vi "VISATCP组合选择发送.vi"(0 "IP":string, 1 "数据发送通道":enum16{"TCP", "VISA"}(ring), 2 "命令":string(combo), 5 "PORT":string, 7 "VISA resource name":refnum<visa-resource-name> caption="VISA资源名称", 9 "baud rate":u32=115200 caption="波特率(115200)", 11 "error in (no error)":errorcluster caption="错误输入（无错误）", 12 "写入缓冲区":string) -> (4 "连接ID":refnum<k5>, 6 "VISA resource name 2":refnum<visa-resource-name>, 13 "读取缓冲区":string, 15 "错误输出":errorcluster)   [LabVIEW 2016, in "数据传输系统-03.lvlib"]
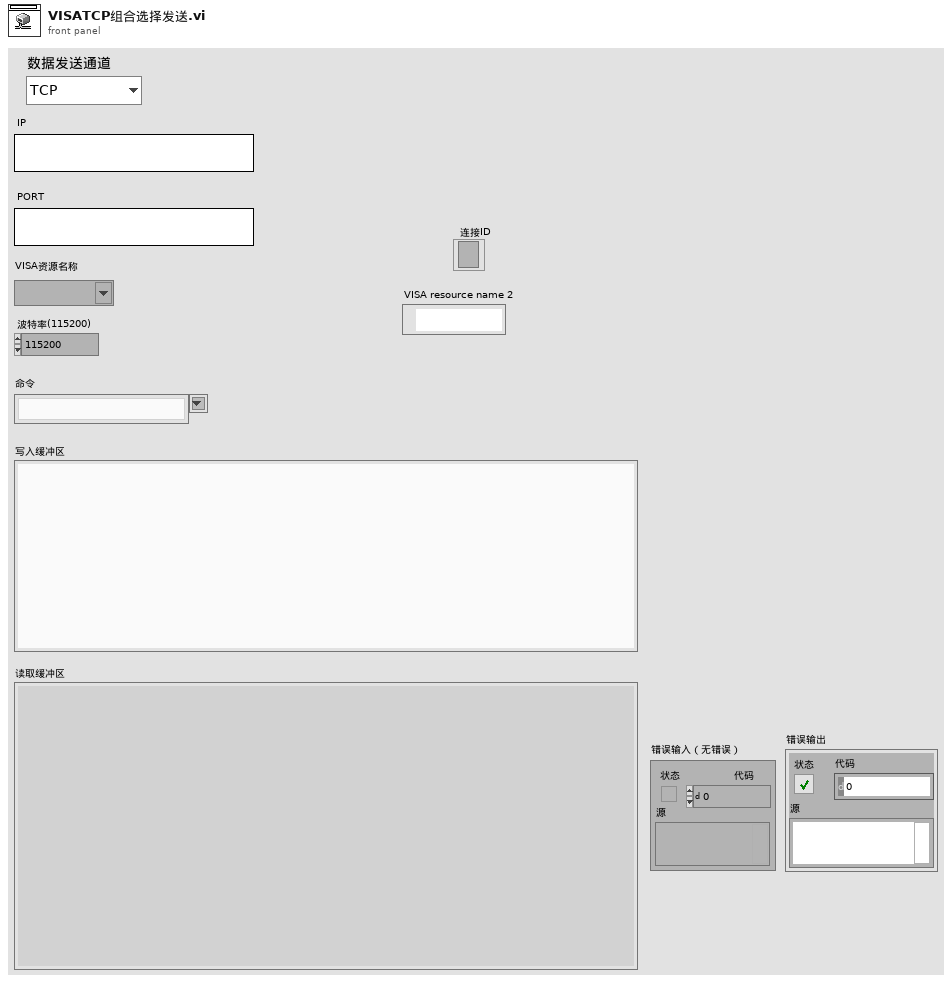
[diagram p1: front panel]
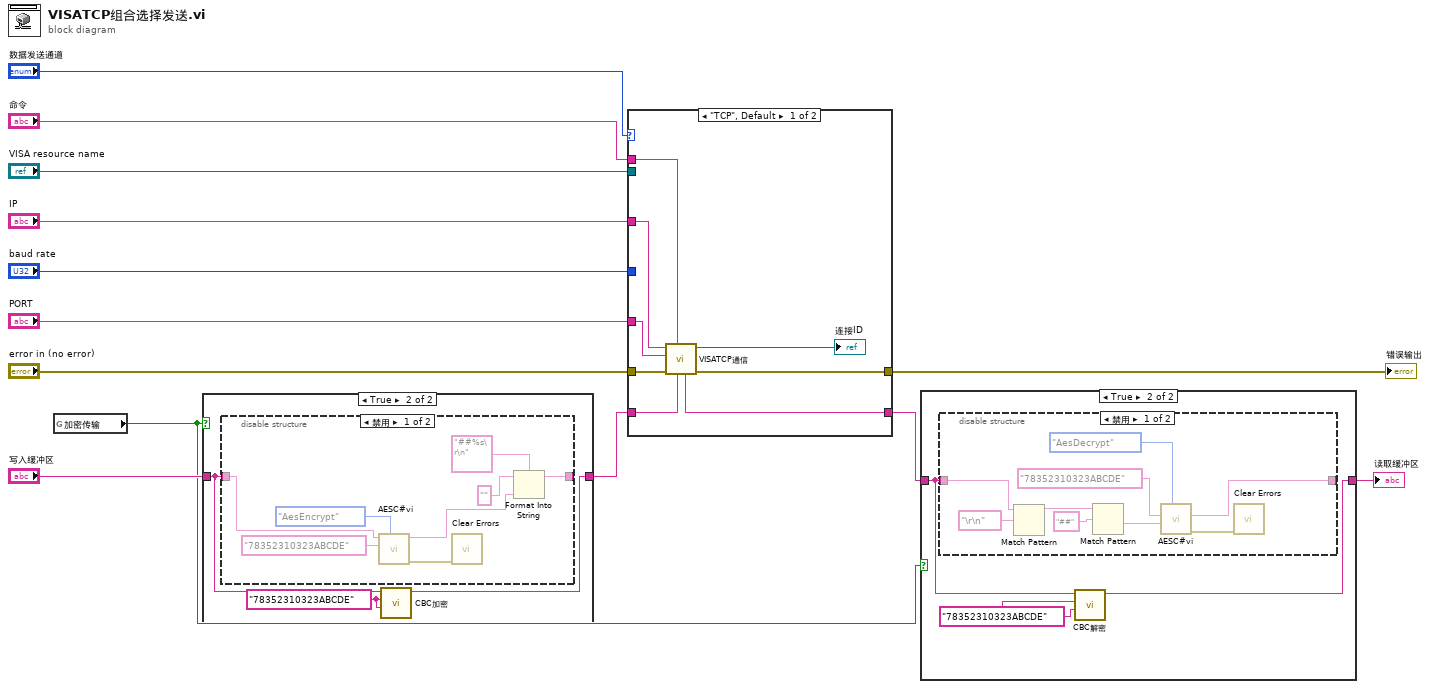
[diagram p0: block diagram]
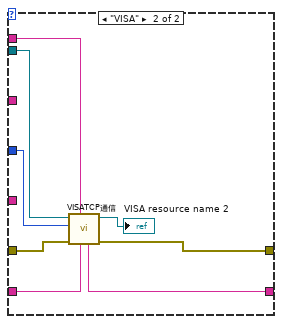
[diagram p6: hidden frame]
diagram:
  n1 = global read "断电保存全局.vi" "加密传输"() -> (w3:bool)
  n2 = case shown="True" w3 {
    tunnel: "写入缓冲区" -> [w14 w17]
    tunnel: [w14 w15] -> w4
    frame False {
    }
    frame True {
      w16 = "78352310323ABCDE" ("钥匙")
      n3 = disable-structure shown="禁用" {
        disable-tunnel: w17 -> [w20 w26]
        disable-tunnel: [w19 w26] -> _
        frame Disabled {
          n4 = call "AESC#vi.vi"("枚举"=enum16{"AesEncrypt", "AesDecrypt"}."AesEncrypt", "key"="78352310323ABCDE", "plainText"=w20) -> ("错误输出"=w18:errorcluster, "AESEncrypt"=w21:string)  [unwired: 6 in, 1 out]
          n5 = call <vilib>:"Clear Errors.vi"("error in (no error)"=w18) -> ()  [unwired: 5 in, 2 out]
          n6 = Format Into String(format string="##%s\r\n", initial string="" ("初始字符串"), w21) -> (resulting string=w19:string)  [unwired: 1 in, 1 out]
        }
        frame Enabled {
        }
      }
      n7 = call "CBC加密.vi"("IV"=w16, "钥匙"=w16, "明文"=w17) -> ("密文"=w15:string)  [unwired: 7 in, 1 out]
    }
  }
  n8 = case shown="\"TCP\", Default" "数据发送通道" {
    tunnel: "命令" -> [w34 w38]
    tunnel: [w33 w40] -> w11
    tunnel: "error in (no error)" -> [w32 w39]
    tunnel: w4 -> [w31 w42]
    tunnel: [w30 w41] -> w2
    tunnel: "PORT" -> [w29 _]
    tunnel: "IP" -> [w28 _]
    tunnel: "baud rate" -> [_ w36]
    tunnel: "VISA resource name" -> [_ w35]
    frame "TCP", Default {
      n9 = call-poly "VISATCP通信.vi"("写入缓冲区"=w31, "命令"=w34, "error in (no error)"=w32, "PORT"=w29, "IP"=w28) -> ("错误输出"=w33:errorcluster, "连接ID"=→"连接ID":refnum<k5>, "读取缓冲区"=w30:string)  [unwired: 4 in]
    }
    frame "VISA" {
      n10 = call-poly "VISATCP通信.vi"("写入缓冲区"=w42, "命令"=w38, "error in (no error)"=w39, "baud rate (9600)"=w36, "VISA resource name"=w35) -> ("错误输出"=w40:errorcluster, "VISA resource name 2"=→"VISA resource name 2":refnum<visa-resource-name>, "读取缓冲区"=w41:string)  [unwired: 4 in]
    }
  }
  "错误输出" <- w11
  n11 = case shown="True" w3 {
    tunnel: w2 -> [w43 w46]
    tunnel: [w43 w44] -> w1
    frame False {
    }
    frame True {
      w45 = "78352310323ABCDE" ("钥匙")
      n12 = disable-structure shown="禁用" {
        disable-tunnel: [w51 w56] -> _
        disable-tunnel: w46 -> [w49 w56]
        frame Disabled {
          n13 = Match Pattern(string=w49, regular expression="\r\n" ("正则表达式")) -> (before substring=w48:string)  [unwired: 1 in, 3 out]
          n14 = Match Pattern(string=w48, regular expression="##" ("正则表达式")) -> (after substring=w47:string)  [unwired: 1 in, 3 out]
          n15 = call "AESC#vi.vi"("枚举"=enum16{"AesEncrypt", "AesDecrypt"}."AesDecrypt", "encryptStr"=w47, "key"="78352310323ABCDE") -> ("错误输出"=w50:errorcluster, "AESDecrypt"=w51:string)  [unwired: 6 in, 1 out]
          n16 = call <vilib>:"Clear Errors.vi"("error in (no error)"=w50) -> ()  [unwired: 5 in, 2 out]
        }
        frame Enabled {
        }
      }
      n17 = call "CBC解密.vi"("IV"=w45, "钥匙"=w45, "密文 in"=w46) -> ("明文"=w44:string)  [unwired: 7 in, 1 out]
    }
  }
  "读取缓冲区" <- w1
